vi "Prepare Without Sniffers.vi"(8 "error in (no error)":errorcluster, 11 "Stream in":refnum<class "Stream.lvclass">) -> (0 "error out":errorcluster, 3 "Stream out":refnum<class "Stream.lvclass">)   [LabVIEW 2020, in "Stream.lvlib" / "Stream.lvclass"]
uses:
  Stream.lvclass
  Stream.lvclass/Stream.ctl
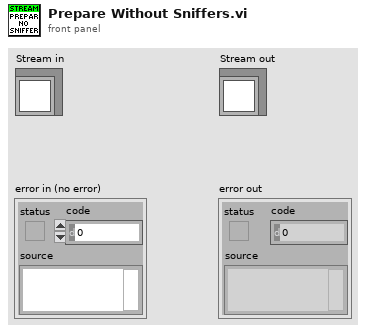
[diagram p1: front panel]
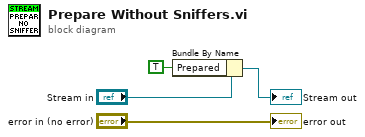
[diagram p0: block diagram]
diagram:
  n1 = Bundle By Name(cluster="Stream in", "Prepared"=TRUE) -> (→"Stream out":refnum<class "Stream.lvclass">)
  "error out" <- "error in (no error)"
